vi "W1DB_Conv_WB2D_int_sub.vi"(1 "Bias":i32, 2 "W_1D":i64[](array[numeric])) -> (0 "2D_WB(29*28)":dbl[][](array[numeric]))   [LabVIEW 2021]
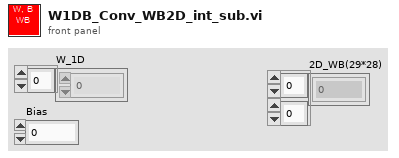
[diagram p1: front panel]
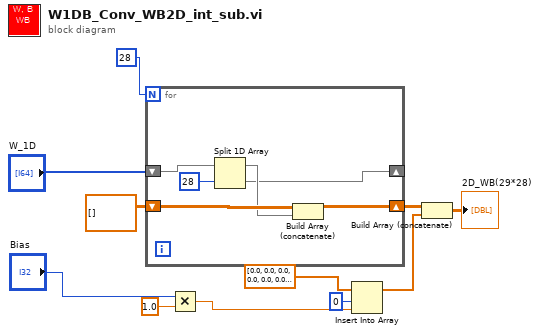
[diagram p0: block diagram]
diagram:
  n1 = for {
    N: 28 -> [_]
    shift-right: [w16] -> w6
    shift-left: dbl[][] [] -> [w15]
    shift-right: [w13] -> _
    shift-left: "W_1D" -> [w12]
    n2 = Split 1D Array(array=w12, index=28) -> (first subarray=w14:i64[], second subarray=w13:i64[])
    n3 = Build Array (concatenate)(w15, w14) -> (w16:dbl[][])
  }
  n4 = Multiply(x="Bias", y=1.0) -> (x*y=w4:dbl)
  n5 = Insert Into Array(array=dbl[] [0.0, 0.0, 0.0, 0.0, 0.0, 0.0, 0.0, 0.0, 0.0, 0.0, 0.0, 0.0, 0.0, 0.0, 0.0, 0.0, 0.0, 0.0, 0.0, 0.0, 0.0, 0.0, 0.0, 0.0, 0.0, 0.0, 0.0] ("두 번째 부분배열"), index=0 ("인덱스"), new element=w4) -> (w7:dbl[])
  n6 = Build Array (concatenate)(w6, w7) -> (→"2D_WB(29*28)":dbl[][])
